vi "Destroy.vi"(0 "reference in":refnum<class "G#RemoteProxy.lvclass">, 5 "error in (no error)":errorcluster) -> (14 "reference out":refnum<class "G#RemoteProxy.lvclass">, 19 "error out":errorcluster)   [LabVIEW 2017, in "G#RemoteProxy.lvclass"]
doc: "Destructor."
uses:
  G#RemoteProxy.lvclass
  G#DebugServer/utils/TCPCommand.ctl
  G#Object/G#Object.lvclass
  G#DebugServer/G#DebugServer.lvclass
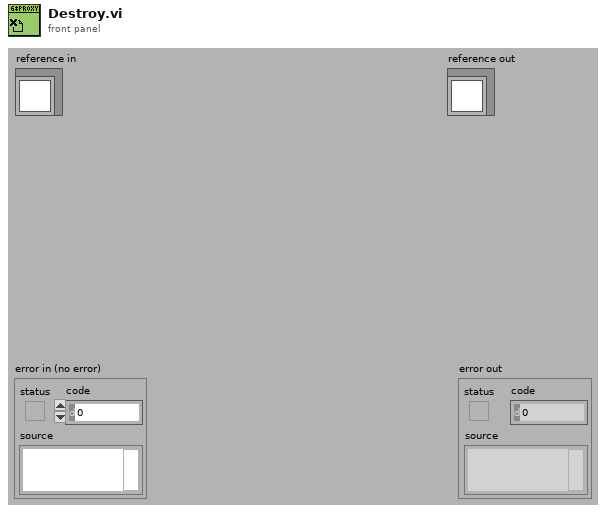
[diagram p1: front panel]
types:
  T1 = typedef "G#RemoteProxy.lvclass/ObjectAttributesProxy.ctl" = cluster{"class hierarchy":T2[], "class name":string, "lvlib hierarchy":string[], "full class name":string, "id":u32, "owner":string, "RemoteRef":refnum<class "G#Object.lvclass">, "object name":string, "attributes":variant[], "connection ID":refnum<k5>, "address":u32, "occurrence":refnum<k4>, "ProxyClassRef":refnum<class "G#RemoteProxy.lvclass">, "InMemory?":bool, "ToString":string}
  T2 = typedef "G#Object.lvclass/G#Object_ClassHierarchy.ctl" = cluster{"ClassName":string, "FullClassName":string, "ClassPath":path, "IsLeaf":bool}
  T3 = typedef "G#DebugServer.lvclass/TCPCommand.ctl" = u8
  T4 = cluster{"InMemory?":bool, "RemoteRef":refnum<class "G#Object.lvclass">}
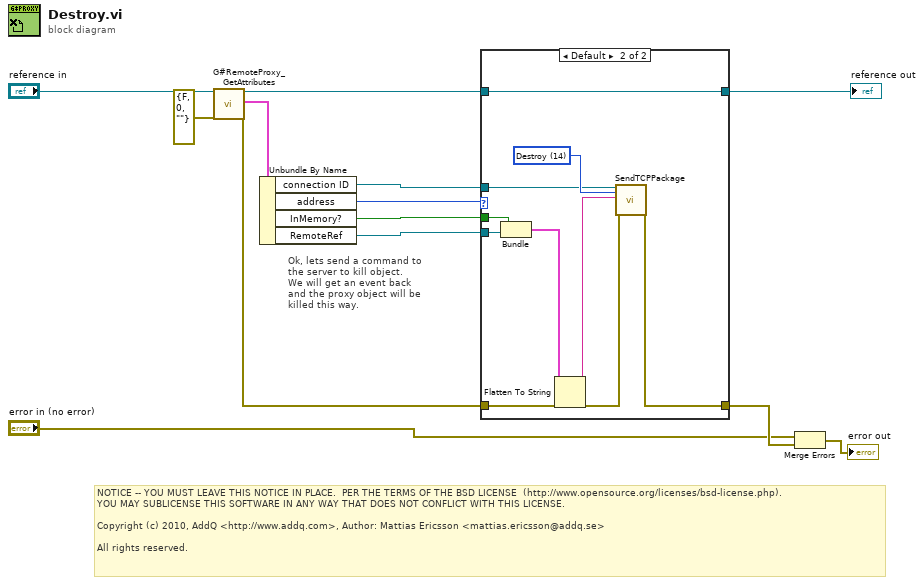
[diagram p0: block diagram]
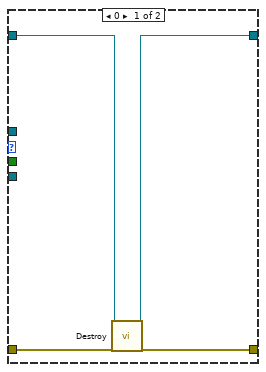
[diagram p2: hidden frame]
diagram:
  # "NOTICE -- YOU MUST LEAVE THIS NOTICE IN PLACE.  PER THE TERMS OF THE BSD LICENSE  (http://www.opensource.org/licenses/bsd-license.php).\nYOU MAY SUBLICENSE THIS SOFTWARE IN ANY WAY THAT DOES NOT CONFLICT WITH THIS LICENSE.\n\nCopyright (c) 2010, AddQ <http://www.addq.com>, Author: Mattias Ericsson <mattias.ericsson@addq.se>\n\nAll rights reserved."
  # "Ok, lets send a command to\nthe server to kill object.\nWe will get an event back\nand the proxy object will be\nkilled this way."
  n1 = call "G#RemoteProxy_GetAttributes.vi"("reference in"="reference in", "error in (no error)"=errorcluster {"status"=FALSE, "code"=0, "source"=""}) -> ("reference out"=w8:refnum<class "G#RemoteProxy.lvclass">, "attributes"=w12:T1, "error out"=w10:errorcluster)  [unwired: 14 in, 1 out]
  n2 = Unbundle By Name(w12) -> ("connection ID"=w11:refnum<k5>, "address"=w9:u32, "InMemory?"=w1:bool, "RemoteRef"=w6:refnum<class "G#Object.lvclass">)
  n3 = case shown="Default" w9 {
    tunnel: w11 -> [_ w18]
    tunnel: w10 -> [w17 w24]
    tunnel: [w16 w27] -> w3
    tunnel: w8 -> [w15 w25]
    tunnel: [w14 w25] -> w7
    tunnel: w6 -> [_ w21]
    tunnel: w1 -> [_ w20]
    frame 0 {
      n4 = call-parent "Destroy.vi"("reference in"=w15, "error in (no error)"=w17) -> ("reference out"=w14:refnum<class "G#RemoteProxy.lvclass">, "error out"=w16:errorcluster)  [unwired: 16 in]
    }
    frame Default {
      w26 = T3 14 items=["GarbageCollect", "GetAllObjects", "GetAllObjectsReply", "CleanUp", "G#Event", "RegisterClient", "GetAttributeValue", "GetAttributeValueReply", "GetClassAttributeValue", "GetClassAttributeValueReply", "GetToStringValue", "GetToStringValueReply", "GetClassHierarchy", "GetClassHierarchyReply", "Destroy"] ("Command")
      n5 = Bundle("InMemory?"=w20, "RemoteRef"=w21) -> (w19:T4)  [unwired: 1 in]
      n6 = Flatten To String(anything=w19, error in (no error)=w24) -> (data string=w22:string, error out=w23:errorcluster)  [unwired: 2 in, 1 out]
      n7 = call "SendTCPPackage.vi"("connection ID"=w18, "command"=w26, "data"=w22, "error in (no error)"=w23) -> ("error out"=w27:errorcluster)  [unwired: 15 in]
    }
  }
  "reference out" <- w7
  n8 = Merge Errors("error in (no error)", w3) -> (→"error out":errorcluster)
